vi "ALL THINGS.vi"() -> ()   [LabVIEW 2018]
panel:
  out "new picture":picture
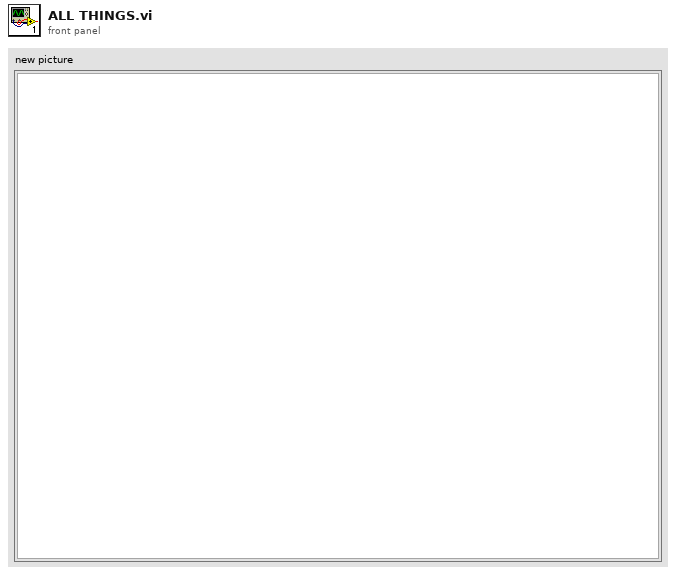
[diagram p1: front panel]
types:
  T1 = typedef "imagedata.ctl" = cluster{"image type":i32, "image depth":i32, "image":u8[], "mask":u8[], "colors":u32[], "Rectangle":cluster{"left":i16, "top":i16, "right":i16, "bottom":i16}}
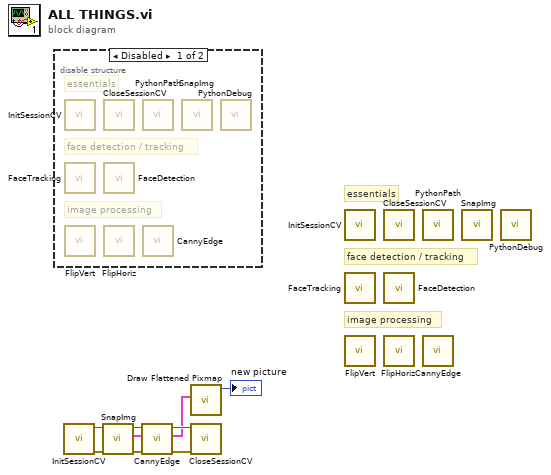
[diagram p0: block diagram]
diagram:
  # "image processing"
  # "face detection / tracking"
  # "essentials"
  n1 = disable-structure shown="Disabled" {
    frame Disabled {
      # "image processing"
      # "face detection / tracking"
      # "essentials"
      n2 = call "InitSessionCV.vi"() -> ()  [unwired: 3 in, 2 out]
      n3 = call "FaceTracking.vi"() -> ()  [unwired: 8 in, 4 out]
      n4 = call "FlipVert.vi"() -> ()  [unwired: 9 in, 3 out]
      n5 = call "CloseSessionCV.vi"() -> ()  [unwired: 4 in]
      n6 = call "FaceDetection.vi"() -> ()  [unwired: 9 in, 3 out]
      n7 = call "FlipHoriz.vi"() -> ()  [unwired: 9 in, 3 out]
      n8 = call "PythonPath.vi"() -> ()  [unwired: 1 out]
      n9 = call "CannyEdge.vi"() -> ()  [unwired: 9 in, 3 out]
      n10 = call "SnapImg.vi"() -> ()  [unwired: 5 in, 3 out]
      n11 = call "PythonDebug.vi"() -> ()  [unwired: 9 in, 3 out]
    }
    frame Enabled {
    }
  }
  n12 = call "InitSessionCV.vi"() -> ("session out"=w9:refnum<k35>, "error out"=w8:errorcluster)  [unwired: 3 in]
  n13 = call "SnapImg.vi"("error in (no error)"=w8, "session in"=w9) -> ("error out"=w7:errorcluster, "img out"=w5:T1, "session out"=w6:refnum<k35>)  [unwired: 3 in]
  n14 = call "CannyEdge.vi"("error in (no error)"=w7, "img in"=w5, "session in"=w6) -> ("error out"=w3:errorcluster, "img out"=w2:T1, "session out"=w4:refnum<k35>)  [unwired: 6 in]
  n15 = call <vilib>:"Draw Flattened Pixmap.vi"("image data"=w2) -> ("new picture"=→"new picture":picture)  [unwired: 8 in]
  n16 = call "CloseSessionCV.vi"("error in (no error)"=w3, "Refnum in"=w4) -> ()  [unwired: 2 in]
  n17 = call "InitSessionCV.vi"() -> ()  [unwired: 3 in, 2 out]
  n18 = call "FaceTracking.vi"() -> ()  [unwired: 8 in, 4 out]
  n19 = call "FlipVert.vi"() -> ()  [unwired: 9 in, 3 out]
  n20 = call "CloseSessionCV.vi"() -> ()  [unwired: 4 in]
  n21 = call "FaceDetection.vi"() -> ()  [unwired: 9 in, 3 out]
  n22 = call "FlipHoriz.vi"() -> ()  [unwired: 9 in, 3 out]
  n23 = call "PythonPath.vi"() -> ()  [unwired: 1 out]
  n24 = call "CannyEdge.vi"() -> ()  [unwired: 9 in, 3 out]
  n25 = call "SnapImg.vi"() -> ()  [unwired: 5 in, 3 out]
  n26 = call "PythonDebug.vi"() -> ()  [unwired: 9 in, 3 out]
